vi "Drive_to_Roll.vi"(1 "Timeout (ms)":dbl, 2 "Roll Cutoff (degrees)":dbl, 3 "Speed (RPM)":dbl) -> ()   [LabVIEW 2020]
uses:
  <vilib>/Rock Robotics/WPI/ThirdParty/REV Robotics/REVLib/Typedef/Spark MAX Control Type.ctl
  <vilib>/Rock Robotics/WPI/ThirdParty/Phoenix-LabVIEW/Pigeon IMU/CTRE_PigeonIMU_GetYPR.vi
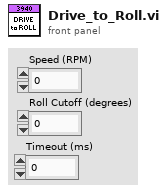
[diagram p1: front panel]
types:
  T1 = typedef "Spark MAX Control Type.ctl" = enum16{"Percent VBus", "Voltage", "Velocity", "Position", "Smart Motion", "Current", "Smart Velocity"}
  T2 = cluster{"P Gain":dbl, "I Gain":dbl, "D Gain":dbl, "F Gain":dbl, "I Zone":dbl, "Min Output":dbl, "Max Output":dbl}
  T3 = typedef "WPI_MotorControlDeviceRef.ctl" = cluster{"DeviceStatus":errorcluster, "Type":T4, "PWM":cluster{"PWM Channel":T5, "DeadBand":T6}, "CAN":cluster{"Device Number":u8, "SetOutput VI Ref":variant, "GetOutput VI Ref":variant, "Enable VI Ref":variant, "Disable VI Ref":variant, "Data":variant}, "Invert":bool, "DIO PWM":cluster{"PWM \"Enable\" Channel":T5, "DIOChannel":T7, "PWM Rate":dbl}}
  T4 = typedef "WPI_MotorControlType.ctl" = enum16{"PWM", "CAN", "DIO PWM"}
  T5 = typedef "FPGA_DIOPWMChannel.ctl" = enum8{"PWM 0", "PWM 1", "PWM 2", "PWM 3", "PWM 4", "PWM 5", "PWM 6", "PWM 7", "PWM 8", "PWM 9", "PWM MXP 0", "PWM MXP 1", "PWM MXP 2", "PWM MXP 3", "PWM MXP 4", "PWM MXP 5", "PWM MXP 6", "PWM MXP 7", "PWM MXP 8", "PWM MXP 9", "Invalid"}
  T6 = typedef "WPI_PWMDeadband.ctl" = cluster{"Name":string, "maxPositivePwm":i32, "minPositivePwm":i32, "centerPwm":i32, "maxNegativePwm":i32, "minNegativePwm":i32, "angularRange":u16}
  T7 = typedef "FPGA_DIOChannel.ctl" = enum8{"DIO 0", "DIO 1", "DIO 2", "DIO 3", "DIO 4", "DIO 5", "DIO 6", "DIO 7", "DIO 8", "DIO 9", "DIO MXP 0", "DIO MXP 1", "DIO MXP 2", "DIO MXP 3", "DIO MXP 4", "DIO MXP 5", "DIO MXP 6", "DIO MXP 7", "DIO MXP 8", "DIO MXP 9", "DIO MXP 10", "DIO MXP 11", "DIO MXP 12", "DIO MXP 13", "DIO MXP 14", "DIO MXP 15", "SPI Port CS1", "SPI Port CS2", "SPI Port CS3", "SPI Port MISO", "SPI Port MOSI", "Invalid"}
  T8 = typedef "CTRE_PigeonIMU_DeviceRef.ctl" = cluster{"DeviceStatus":errorcluster, "Device Number":u8, "Type":T9, "Device ID":u32, "Handle":u64, "UsageFrame":u32, "Library Path":path}
  T9 = typedef "CTRE_PigeonIMU_ConnectionType.ctl" = u32
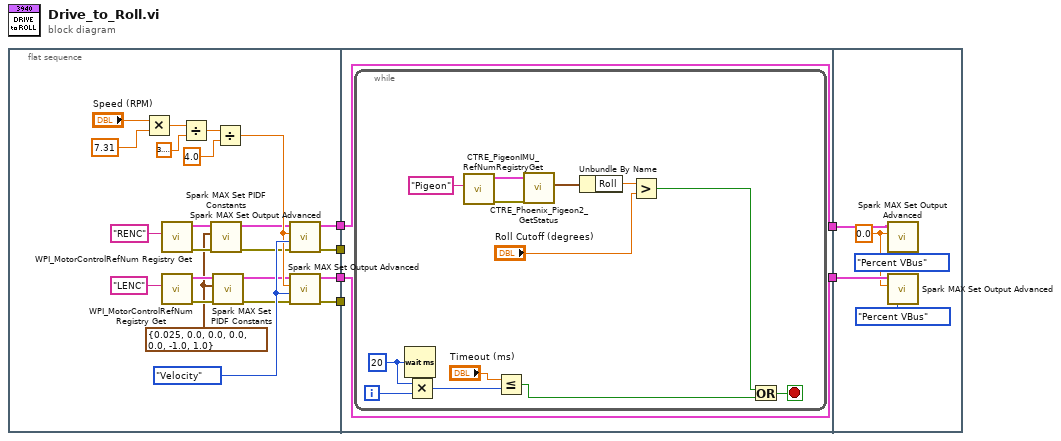
[diagram p0: block diagram]
diagram:
  n1 = flat-sequence {
    tunnel: [w15] -> w6
    tunnel: [w14] -> w5
    tunnel: [w13] -> w4
    tunnel: [w12] -> w3
    tunnel: w6 -> [w31]
    tunnel: w5 -> [w30]
    tunnel: w4 -> [_]
    tunnel: w3 -> [_]
    tunnel: [w31] -> w2
    tunnel: [w30] -> w1
    tunnel: w2 -> [w49]
    tunnel: w1 -> [w48]
    frame #0 {
      w22 = Spark_MAX_Control_Type."Velocity" ("Control Mode")
      w23 = T2 {"P Gain"=0.025, "I Gain"=0.0, "D Gain"=0.0, "F Gain"=0.0, "I Zone"=0.0, "Min Output"=-1.0, "Max Output"=1.0} ("PID Constants")
      n2 = Multiply(x="Speed (RPM)", y=7.31) -> (x*y=w20:dbl)
      n3 = call <vilib>:"WPI_MotorControlRefNum Registry Get.vi"("refnum name"="RENC") -> ("error out"=w27:errorcluster, "MotorControlDevRef"=w26:T3)  [unwired: 9 in]
      n4 = call <vilib>:"WPI_MotorControlRefNum Registry Get.vi"("refnum name"="LENC") -> ("error out"=w25:errorcluster, "MotorControlDevRef"=w24:T3)  [unwired: 9 in]
      n5 = Divide(x=w20, y=3.141592653589793) -> (x/y=w18:dbl)
      n6 = call <vilib>:"Spark MAX Set PIDF Constants.vi"("error in"=w27, "PID Constants"=w23, "MotorControlDeviceRef"=w26) -> ("error out"=w7:errorcluster, "MotorControlDeviceRef"=w10:T3)  [unwired: 7 in]
      n7 = call <vilib>:"Spark MAX Set PIDF Constants.vi"("error in"=w25, "PID Constants"=w23, "MotorControlDeviceRef"=w24) -> ("error out"=w8:errorcluster, "MotorControlDeviceRef"=w9:T3)  [unwired: 7 in]
      n8 = Divide(x=w18, y=4.0) -> (x/y=w16:dbl)
      n9 = call <vilib>:"Spark MAX Set Output Advanced.vi"("error in (no error)"=w7, "Control Mode"=w22, "Setpoint"=w16, "MotorControlDevRef"=w10) -> ("error out"=w12:errorcluster, "MotorControlDevRef"=w15:T3)  [unwired: 6 in]
      n10 = call <vilib>:"Spark MAX Set Output Advanced.vi"("error in (no error)"=w8, "Control Mode"=w22, "Setpoint"=w16, "MotorControlDevRef"=w9) -> ("error out"=w13:errorcluster, "MotorControlDevRef"=w14:T3)  [unwired: 6 in]
    }
    frame #1 {
      n11 = while {
        i -> [w44]
        stop <- w39 stop-if-true
        w43 = u32 20 ("milliseconds to wait")
        n12 = Wait (ms)(milliseconds to wait=w43) -> ()  [unwired: 1 out]
        n13 = Multiply(x=w43, y=w44) -> (x*y=w42:u32)
        n14 = call <vilib>:"CTRE_PigeonIMU_RefNumRegistryGet.vi"("refnum name"="Pigeon") -> ("error out"=w38:errorcluster, "PigeonIMUDevRef"=w37:T8)  [unwired: 9 in]
        n15 = Less Or Equal?(x="Timeout (ms)", y=w42) -> (x <= y?=w40:bool)
        n16 = call-poly <vilib>:"CTRE_Phoenix_Pigeon2_GetStatus.vi"("error in (no error)"=w38, "PigeonIMUDevRef"=w37) -> ("Yaw Pitch Roll"=w35:cluster{"Yaw":dbl, "Pitch":dbl, "Roll":dbl})  [unwired: 7 in, 2 out]
        n17 = Unbundle By Name(w35) -> ("Roll"=w34:dbl)
        n18 = Greater?(x=w34, y="Roll Cutoff (degrees)") -> (0:w32:bool)
        n19 = Or(x=w32, y=w40) -> (x .or. y?=w39:bool)
      }
    }
    frame #2 {
      w47 = 0.0 ("Setpoint")
      n20 = call <vilib>:"Spark MAX Set Output Advanced.vi"("Control Mode"=Spark_MAX_Control_Type."Percent VBus", "Setpoint"=w47, "MotorControlDevRef"=w49) -> ()  [unwired: 7 in, 2 out]
      n21 = call <vilib>:"Spark MAX Set Output Advanced.vi"("Control Mode"=Spark_MAX_Control_Type."Percent VBus", "Setpoint"=w47, "MotorControlDevRef"=w48) -> ()  [unwired: 7 in, 2 out]
    }
  }
